vi "GetDetails.vi"(8 "error in (no error)":errorcluster, 11 "reference in":refnum<class "ViPER.lvclass">) -> (0 "error out":errorcluster, 2 "Details":T1, 3 "reference out":refnum<class "ViPER.lvclass">)   [LabVIEW 2022 SP3, in "ViPER.lvlib" / "ViPER.lvclass"]
uses:
  ViPER.lvclass
  Version.ctl
  <userlib>/_OpenG.lib/md5/md5.llb/MD5 Message Digest (Hexadecimal String)__ogtk.vi
panel:
  # "### BSD License (http://www.opensource.org/licenses/bsd-license.php) Begin ###\n\nCopyright (c) 2018  Kurt Friday www.medulla.net\n\nAll rights reserved.\n\nRedistribution and use in source and binary forms, with or without\nmodification, are permitted provided that the following conditions are met:\n\n    * Redistributions of source code must retain the above copyright\n      notice, this list of conditions and the following disclaimer.\n\n    * Redistributions in binary form must reproduce the above copyright\n      notice, this list of conditions and the following disclaimer in the\n      documentation and/or other materials provided with the distribution.\n\n    * Neither the name of the <organization> nor the\n      names of its contributors may be used to endorse or promote products\n      derived from this software without specific prior written permission.\n\nTHIS SOFTWARE IS PROVIDED BY THE COPYRIGHT HOLDERS AND CONTRIBUTORS \"AS IS\" AND\nANY EXPRESS OR IMPLIED WARRANTIES, INCLUDING, BUT NOT LIMITED TO, THE IMPLIED\nWARRANTIES OF MERCHANTABILITY AND FITNESS FOR A PARTICULAR PURPOSE ARE\nDISCLAIMED. IN NO EVENT SHALL <COPYRIGHT HOLDER> BE LIABLE FOR ANY\nDIRECT, INDIRECT, INCIDENTAL, SPECIAL, EXEMPLARY, OR CONSEQUENTIAL DAMAGES\n(INCLUDING, BUT NOT LIMITED TO, PROCUREMENT OF SUBSTITUTE GOODS OR SERVICES;\nLOSS OF USE, DATA, OR PROFITS; OR BUSINESS INTERRUPTION) HOWEVER CAUSED AND\nON ANY THEORY OF LIABILITY, WHETHER IN CONTRACT, STRICT LIABILITY, OR TORT\n(INCLUDING NEGLIGENCE OR OTHERWISE) ARISING IN ANY WAY OUT OF THE USE OF THIS\nSOFTWARE, EVEN IF ADVISED OF THE POSSIBILITY OF SUCH DAMAGE."
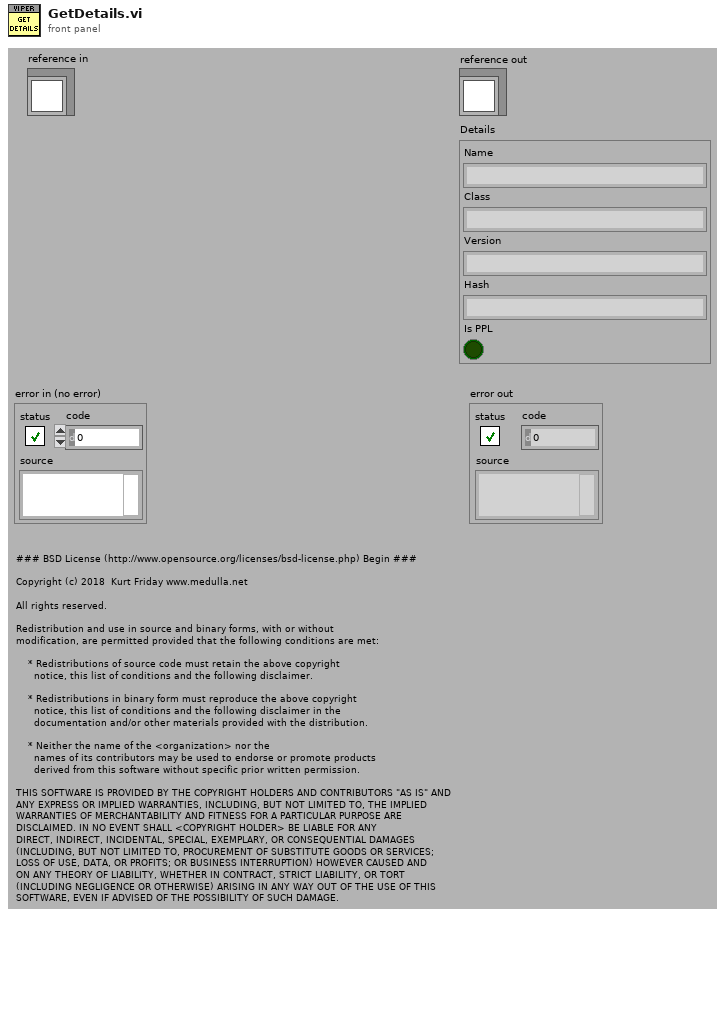
[diagram p1: front panel]
types:
  T1 = typedef "ViPER.lvlib/ViPER.lvclass/Version.ctl" = cluster{"Name":string, "Class":string, "Version":string, "Hash":string, "Is PPL":bool}
  T2 = typedef "ViPER.lvlib/ViPER.lvclass/Details.ctl" = cluster{"Name":string, "Class":string}
  T3 = typedef "ViPER.lvlib/ViPER.lvclass/ObjectAttributes.ctl" = cluster{"Object":T4, "Ancestors":T6[], "Config":T7, "Init_OK":bool, "Hierachy":string[], "PPL?":bool[], "SFP_Open":bool[], "Config_SFP_Open":bool[], "SoftFP_event":refnum<user-event>[], "ConfigFP_event":refnum<user-event>[], "SoftFP_Shutdown_Notifier":refnum<notifier>[], "ConfigFP_Shutdown_Notifier":refnum<notifier>[]}
  T4 = typedef "ViPER.lvlib/ViPER.lvclass/ObjectDefinition.ctl" = cluster{"Name":string, "Ancestors":T5[]}
  T5 = typedef "ViPER.lvlib/ViPER.lvclass/Ancestor.ctl" = cluster{"Class":string, "Config":string, "Objects":string[]}
  T6 = typedef "ViPER.lvlib/ViPER.lvclass/ObjectLayers.ctl" = cluster{"Ancestor":string, "Objects":refnum<class "ViPER.lvclass">[], "Object_Names":string[], "Owned":bool[]}
  T7 = typedef "ViPER.lvlib/ViPER.lvclass/Config.ctl" = cluster{"default":string}
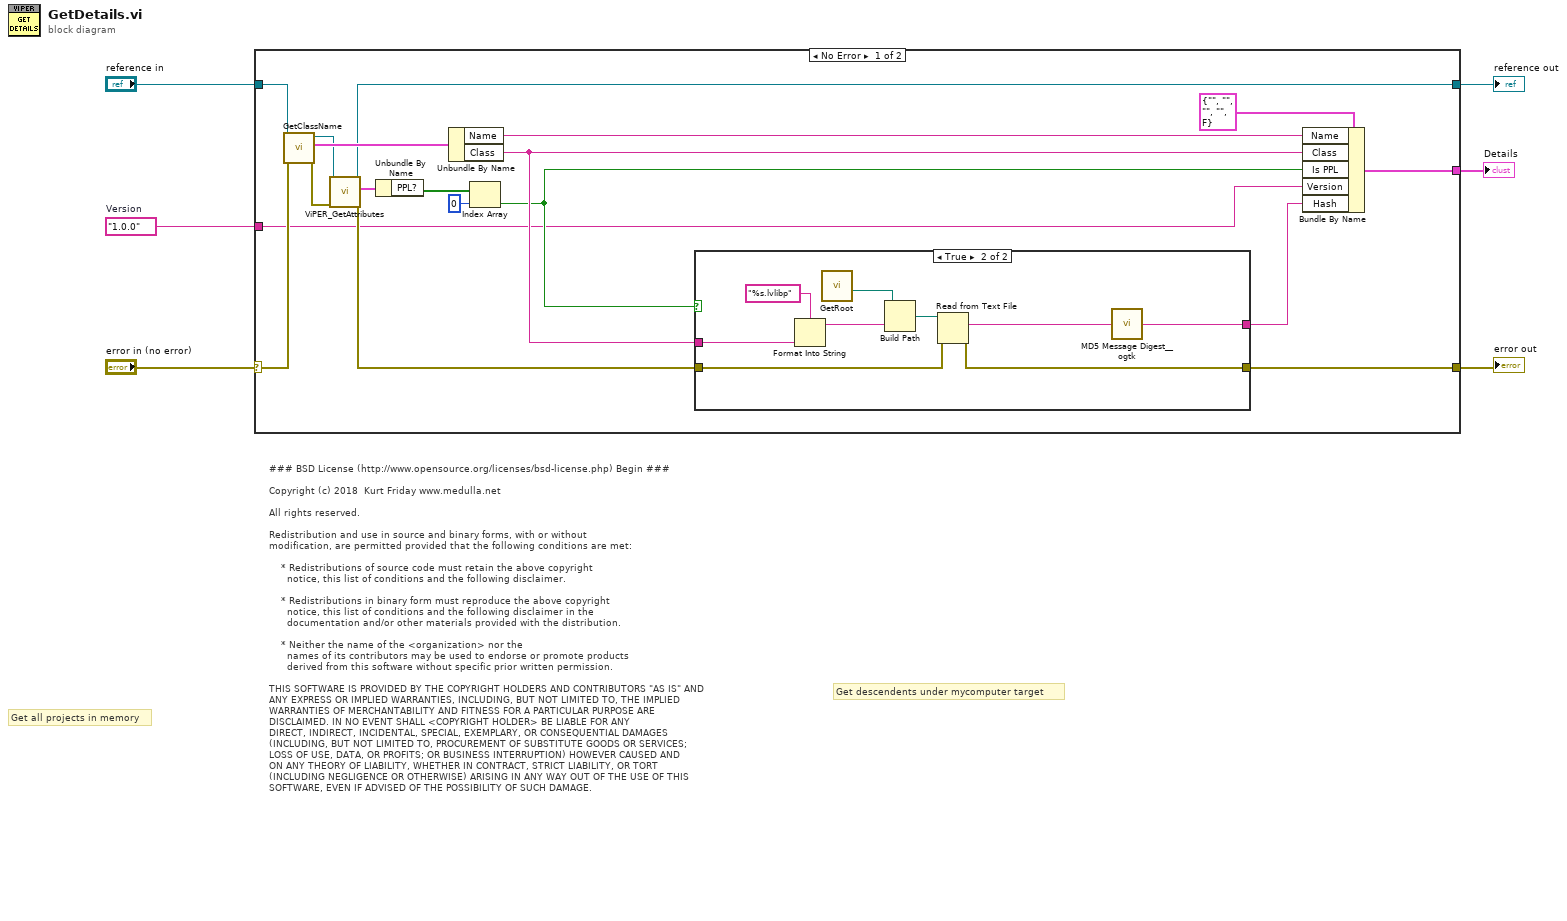
[diagram p0: block diagram]
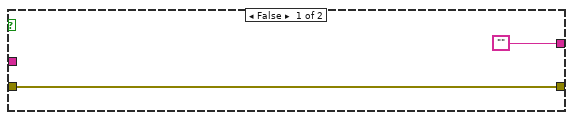
[diagram p2: hidden frame]
diagram:
  w1 = "1.0.0"  # Version
  # "### BSD License (http://www.opensource.org/licenses/bsd-license.php) Begin ###\n\nCopyright (c) 2018  Kurt Friday www.medulla.net\n\nAll rights reserved.\n\nRedistribution and use in source and binary forms, with or without\nmodification, are permitted provided that the following conditions are met:\n\n    * Redistributions of source code must retain the above copyright\n      notice, this list of conditions and the following disclaimer.\n\n    * Redistributions in binary form must reproduce the above copyright\n      notice, this list of conditions and the following disclaimer in the\n      documentation and/or other materials provided with the distribution.\n\n    * Neither the name of the <organization> nor the\n      names of its contributors may be used to endorse or promote products\n      derived from this software without specific prior written permission.\n\nTHIS SOFTWARE IS PROVIDED BY THE COPYRIGHT HOLDERS AND CONTRIBUTORS \"AS IS\" AND\nANY EXPRESS OR IMPLIED WARRANTIES, INCLUDING, BUT NOT LIMITED TO, THE IMPLIED\nWARRANTIES OF MERCHANTABILITY AND FITNESS FOR A PARTICULAR PURPOSE ARE\nDISCLAIMED. IN NO EVENT SHALL <COPYRIGHT HOLDER> BE LIABLE FOR ANY\nDIRECT, INDIRECT, INCIDENTAL, SPECIAL, EXEMPLARY, OR CONSEQUENTIAL DAMAGES\n(INCLUDING, BUT NOT LIMITED TO, PROCUREMENT OF SUBSTITUTE GOODS OR SERVICES;\nLOSS OF USE, DATA, OR PROFITS; OR BUSINESS INTERRUPTION) HOWEVER CAUSED AND\nON ANY THEORY OF LIABILITY, WHETHER IN CONTRACT, STRICT LIABILITY, OR TORT\n(INCLUDING NEGLIGENCE OR OTHERWISE) ARISING IN ANY WAY OUT OF THE USE OF THIS\nSOFTWARE, EVEN IF ADVISED OF THE POSSIBILITY OF SUCH DAMAGE."
  # "Get descendents under mycomputer target"
  # "Get all projects in memory"
  n1 = case shown="No Error" "error in (no error)" {
    selector: "error in (no error)" -> [w22 w37]
    tunnel: [w24 w37] -> w4
    tunnel: [w14 w36] -> w3
    tunnel: "reference in" -> [w21 w36]
    tunnel: [w16 _] -> w2
    tunnel: w1 -> [w7 _]
    frame No Error {
      n2 = call "GetClassName.vi"("error in (no error)"=w22, "reference in"=w21) -> ("error out"=w13:errorcluster, "Details"=w23:T2, "reference out"=w15:refnum<class "ViPER.lvclass">)  [unwired: 7 in]
      n3 = call "ViPER_GetAttributes.vi"("error in (no error)"=w13, "reference in"=w15) -> ("error out"=w8:errorcluster, "Data"=w12:T3, "reference out"=w14:refnum<class "ViPER.lvclass">)  [unwired: 6 in, 1 out]
      n4 = Unbundle By Name(w12) -> ("PPL?"=w11:bool[])
      n5 = Unbundle By Name(w23) -> ("Name"=w19:string, "Class"=w18:string)
      n6 = Index Array(array=w11, index=0) -> (element=w9:bool)
      n7 = case shown="True" w9 {
        tunnel: [w26 w30] -> w24
        tunnel: w8 -> [w26 w31]
        tunnel: w18 -> [_ w33]
        tunnel: ["" w27] -> w17
        frame False {
        }
        frame True {
          n8 = Format Into String(format string="%s.lvlibp", w33) -> (resulting string=w34:string)  [unwired: 2 in, 1 out]
          n9 = call "GetRoot.vi"() -> ("Root"=w32:path)  [unwired: 10 in, 1 out]
          n10 = Build Path(base path=w32, name or relative path=w34) -> (appended path=w29:path)
          n11 = Read from Text File(file (use dialog)=w29, error in=w31) -> (text=w28:string, error out=w30:errorcluster)  [unwired: 2 in, 2 out]
          n12 = call-poly <userlib>:"MD5 Message Digest__ogtk.vi"("Message"=w28) -> ("MD5 Message Digest"=w27:string)
        }
      }
      n13 = Bundle By Name(cluster=T1 {"Name"="", "Class"="", "Version"="", "Hash"="", "Is PPL"=FALSE} ("Object Version Info"), "Name"=w19, "Class"=w18, "Is PPL"=w9, "Version"=w7, "Hash"=w17) -> (w16:T1)
    }
    frame Error {
    }
  }
  "error out" <- w4
  "reference out" <- w3
  "Details" <- w2
